vi "Write VNA ports.vi"(10 "VNA ports":bool[](array[boolean])=[TRUE, FALSE, FALSE, FALSE], 11 "S Parameter in":refnum<class "S Parameter.lvclass">) -> (3 "S Parameter out":refnum<class "S Parameter.lvclass">)   [LabVIEW 2020, in "S Parameter.lvclass"]
uses:
  S Parameter.lvclass
  S Parameter.lvclass/S Parameter.ctl
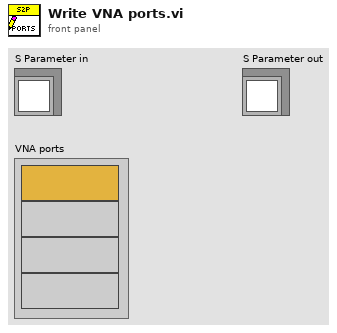
[diagram p1: front panel]
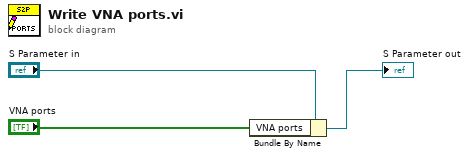
[diagram p0: block diagram]
diagram:
  n1 = Bundle By Name(cluster="S Parameter in", "VNA ports"="VNA ports") -> (→"S Parameter out":refnum<class "S Parameter.lvclass">)
